vi "PrintLibraryToHTML.vi"(3 "outputFolder":path=path "C:/Users/dallis/OneDrive - Velico Medical/Documents/Personal/LabVIEW Coding Projects/Lumberjack/docs/HTMLReport", 8 "error in (no error)":errorcluster, 11 "sourcePaths":path[](array[path])=[path "C:/Users/dallis/OneDrive - Velico Medical/Documents/Personal/LabVIEW Coding Projects/Lumberjack/src", path "C:/Users/dallis/OneDrive - Velico Medical/Documents/Personal/LabVIEW Coding Projects/Lumberjack/tests"]) -> (0 "error out":errorcluster)   [LabVIEW 2026]
uses:
  <vilib>/Utility/miscctls.llb/LVPointTypeDef.ctl
  <vilib>/AdvancedString/Delimited String to 1D String Array (string).vi
  <vilib>/AdvancedString/1D String Array to Delimited String (string).vi
panel:
  out "Array":path[](array[path])
  in  "Individual Files?":bool
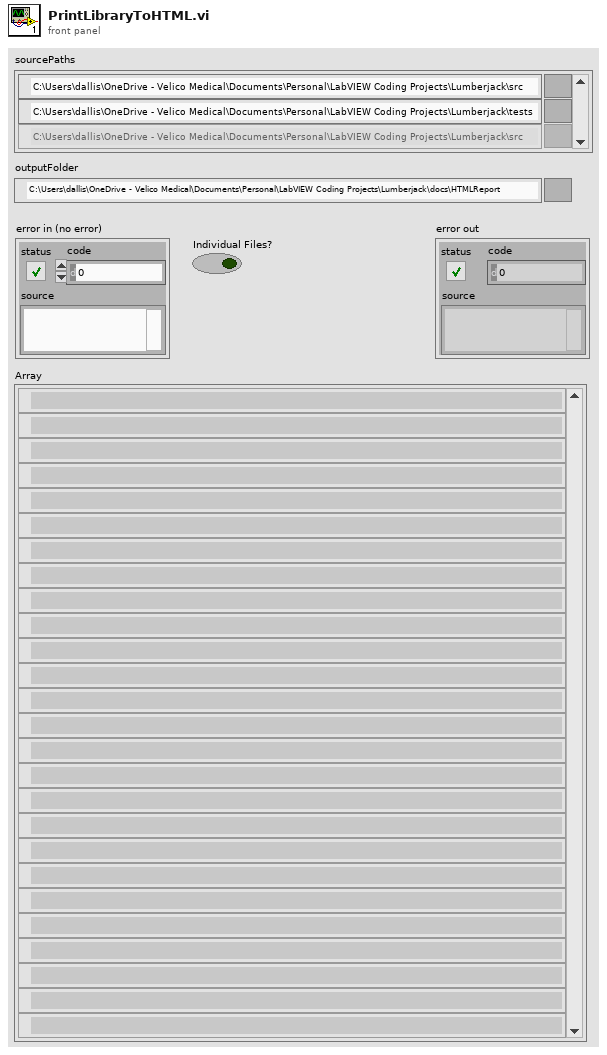
[diagram p1: front panel]
types:
  T1 = typedef "LVPointTypeDef.ctl" = cluster{"Horizontal":i16, "Vertical":i16}
  T2 = enum32{"Custom", "Standard", "Using Panel", "Using SubVI", "Complete"}
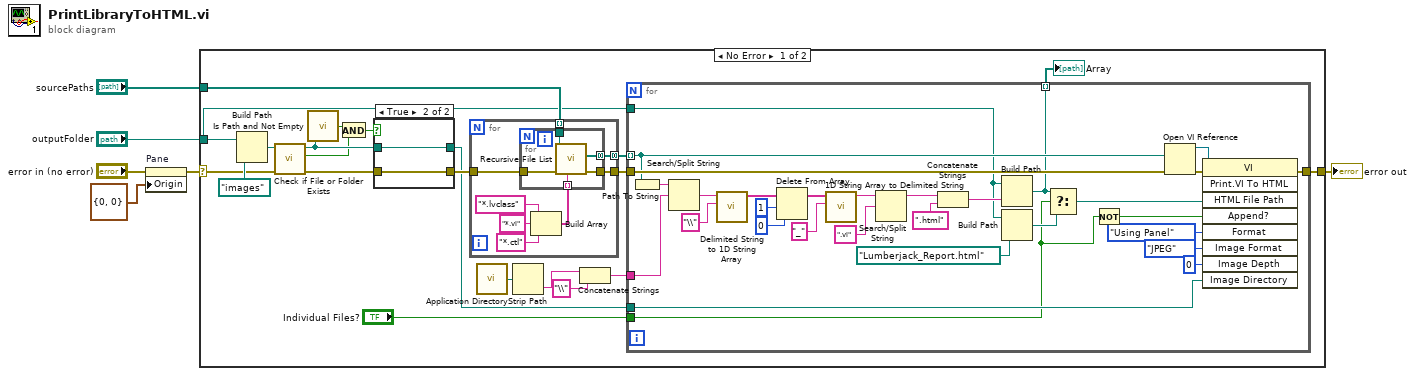
[diagram p0: block diagram]
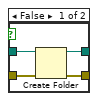
[diagram p2: hidden frame]
diagram:
  n1 = property on="Pane" class="Pane"(error in="error in (no error)", "Origin"=T1 {"Horizontal"=0, "Vertical"=0}) -> (error out=w3:errorcluster)  [unwired: 1 in, 1 out]
  n2 = case shown="No Error" w3 {
    selector: w3 -> [w26 w77]
    tunnel: [w15 w77] -> w6
    tunnel: "sourcePaths" -> [w16 _]
    tunnel: "outputFolder" -> [w13 _]
    frame No Error {
      n3 = Build Path(base path=w13, name or relative path=path "images") -> (appended path=w25:path)
      n4 = call <vilib>:"Check if File or Folder Exists.vi"("error in (no error)"=w26, "path"=w25) -> ("error out"=w23:errorcluster, "file or folder exists?"=w21:bool, "dup path"=w24:path)  [unwired: 7 in]
      n5 = call <vilib>:"Is Path and Not Empty.vi"("path"=w24) -> ("Is Path and Not Empty?"=w22:bool)  [unwired: 4 in]
      n6 = And(x=w22, y=w21) -> (x .and. y?=w20:bool)
      n7 = case shown="True" w20 {
        tunnel: w24 -> [w74 w76]
        tunnel: w23 -> [w73 w75]
        tunnel: [w72 w75] -> w19
        tunnel: [w71 w76] -> w17
        frame False {
          n8 = Create Folder(path (use dialog)=w74, error in=w73) -> (created path=w71:path, error out=w72:errorcluster)  [unwired: 1 in, 1 out]
        }
        frame True {
        }
      }
      n9 = for {
        tunnel: [w34] -> w11 mode=concatenating
        tunnel: w16 -> [w32] mode=indexing
        tunnel: w19 -> [w35]
        tunnel: [w33] -> w18
        n10 = Build Array("*.lvclass" ("pattern"), "*.vi" ("pattern"), "*.ctl" ("pattern")) -> (w29:string[])
        n11 = for {
          tunnel: [w39] -> w34 mode=concatenating
          tunnel: w32 -> [w37]
          tunnel: w29 -> [w36] mode=indexing
          tunnel: w35 -> [w40]
          tunnel: [w38] -> w33
          n12 = call <vilib>:"Recursive File List.vi"("pattern"=w36, "error in (no error)"=w40, "Folder Path"=w37) -> ("error out"=w38:errorcluster, "All Files in Dir"=w39:path[])  [unwired: 4 in, 3 out]
        }
      }
      n13 = call <vilib>:"Application Directory.vi"() -> ("Application Directory"=w10:path)
      n14 = Strip Path(path=w10) -> (name=w9:string)  [unwired: 1 out]
      n15 = Concatenate Strings(w9, "\\" ("string")) -> (w7:string)
      n16 = for {
        tunnel: w11 -> [w54] mode=indexing
        tunnel: w13 -> [w43]
        tunnel: w18 -> [w56]
        tunnel: w17 -> [w58]
        tunnel: [w57] -> w15
        tunnel: "Individual Files?" -> [w44]
        tunnel: [w42] -> w12 mode=indexing
        tunnel: w7 -> [w41]
        n17 = Path To String(path=w54) -> (string=w70:string)
        n18 = Search/Split String(string=w70, search string/char (-)=w41) -> (match + rest of string=w69:string)  [unwired: 1 in, 2 out]
        n19 = call-poly <vilib>:"Delimited String to 1D String Array.vi"("delimiter"="\\", "delimited string"=w69) -> ("string array"=w65:string[])  [unwired: 9 in]
        n20 = Delete From Array(array=w65, length=1, index=0) -> (array with subset deleted=w64:string[])  [unwired: 1 out]
        n21 = call-poly <vilib>:"1D String Array to Delimited String.vi"("delimiter"="_" ("element"), "string array"=w64) -> ("delimited string"=w62:string)  [unwired: 9 in]
        n22 = Search/Split String(string=w62, search string/char (-)=".vi") -> (substring before match=w60:string)  [unwired: 1 in, 2 out]
        n23 = Concatenate Strings(w60, ".html" ("element")) -> (w55:string)
        n24 = Build Path(base path=w43, name or relative path=w55) -> (appended path=w42:path)
        n25 = Build Path(base path=w43, name or relative path=path "Lumberjack_Report.html") -> (appended path=w48:path)
        n26 = Select(t=w42, s=w44, f=w48) -> (s? t:f=w47:path)
        n27 = Not(x=w44) -> (.not. x?=w45:bool)
        n28 = Open VI Reference(vi path=w54, error in (no error)=w56) -> (vi reference=w52:refnum<vi>, error out=w53:errorcluster)  [unwired: 4 in]
        n29 = invoke class="VI" method="Print.VI To HTML"(reference=w52, error in=w53, "HTML File Path"=w47, "Append?"=w45, "Format"=T2."Using Panel", "Image Format"=enum32{"PNG", "JPEG", "GIF"}."JPEG", "Image Depth"=0, "Image Directory"=w58) -> (error out=w57:errorcluster)  [unwired: 1 in, 8 out]
      }
      "Array" <- w12
    }
    frame Error {
    }
  }
  "error out" <- w6
